vi "CRYSet Limits Run Front Panel.vi"(11 "Vi Ref":refnum<vi>) -> ()   [LabVIEW 2013]
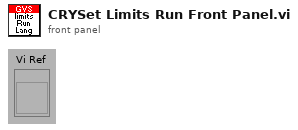
[diagram p1: front panel]
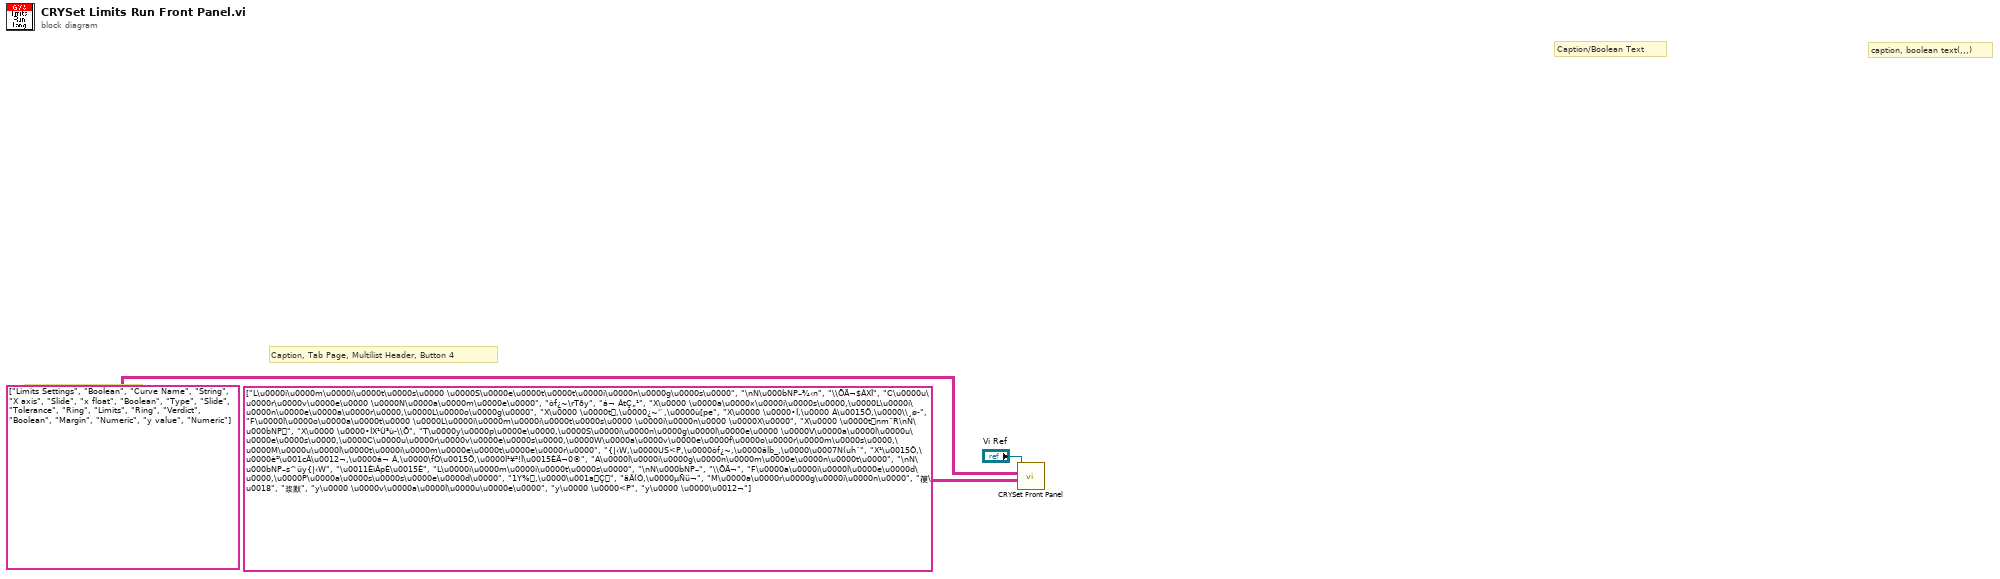
[diagram p0: block diagram]
diagram:
  # "Caption, Tab Page, Multilist Header, Button 4"
  # "Control Type"
  # "Control Name and Tab"
  # "caption, boolean text(,,,)"
  # "Caption/Boolean Text"
  n1 = call "CRYSet Front Panel.vi"("Caption(Boolean Text)"=string[][] [["L\u0000i\u0000m\u0000i\u0000t\u0000s\u0000 \u0000S\u0000e\u0000t\u0000t\u0000i\u0000n\u0000g\u0000s\u0000", "\nN\u000bNP–¾‹n", "\\ÕÄ¬$ÁXÎ"], ["C\u0000u\u0000r\u0000v\u0000e\u0000 \u0000N\u0000a\u0000m\u0000e\u0000", "òf¿~\rTðy", "á¬ ÁtÇ„¹"], ["X\u0000 \u0000a\u0000x\u0000i\u0000s\u0000,\u0000L\u0000i\u0000n\u0000e\u0000a\u0000r\u0000,\u0000L\u0000o\u0000g\u0000", "X\u0000 \u0000t,\u0000¿~'`,\u0000ù[pe", "X\u0000 \u0000•Í,\u0000 Á\u0015Ö,\u0000\\¸ø­"], ["F\u0000l\u0000o\u0000a\u0000t\u0000 \u0000L\u0000i\u0000m\u0000i\u0000t\u0000s\u0000 \u0000i\u0000n\u0000 \u0000X\u0000", "X\u0000 \u0000tnm¨R\nN\u000bNP", "X\u0000 \u0000•ÍX¹Ù³ù­\\Õ"], ["T\u0000y\u0000p\u0000e\u0000,\u0000S\u0000i\u0000n\u0000g\u0000l\u0000e\u0000 \u0000V\u0000a\u0000l\u0000u\u0000e\u0000s\u0000,\u0000C\u0000u\u0000r\u0000v\u0000e\u0000s\u0000,\u0000W\u0000a\u0000v\u0000e\u0000f\u0000o\u0000r\u0000m\u0000s\u0000,\u0000M\u0000u\u0000l\u0000t\u0000i\u0000m\u0000e\u0000t\u0000e\u0000r\u0000", "{|‹W,\u0000US<P,\u0000òf¿~,\u0000âlb_,\u0000\u0007N(uhˆ", "X¹\u0015Ö,\u0000è²\u001cÂ\u0012¬,\u0000á¬ Á,\u0000\fÓ\u0015Ö,\u0000Ì¹¥²!Î\u0015ÈÄ¬0®"], ["A\u0000l\u0000i\u0000g\u0000n\u0000m\u0000e\u0000n\u0000t\u0000", "\nN\u000bNP–s^ûy{|‹W", "\u0011ÉìÂpÈ\u0015È"], ["L\u0000i\u0000m\u0000i\u0000t\u0000s\u0000", "\nN\u000bNP–", "\\ÕÄ¬"], ["F\u0000a\u0000i\u0000l\u0000e\u0000d\u0000,\u0000P\u0000a\u0000s\u0000s\u0000e\u0000d\u0000", "1Y%,\u0000\u001aÇ", "äÂ(Ó,\u0000µÑü¬"], ["M\u0000a\u0000r\u0000g\u0000i\u0000n\u0000", "箯\u0018", "浆默"], ["y\u0000 \u0000v\u0000a\u0000l\u0000u\u0000e\u0000", "y\u0000 \u0000<P", "y\u0000 \u0000\u0012¬"]], "Control ID and Type(Label Name, Type)"=string[][] [["Limits Settings", "Boolean"], ["Curve Name", "String"], ["X axis", "Slide"], ["x float", "Boolean"], ["Type", "Slide"], ["Tolerance", "Ring"], ["Limits", "Ring"], ["Verdict", "Boolean"], ["Margin", "Numeric"], ["y value", "Numeric"]], "Vi Ref"="Vi Ref") -> ()  [unwired: 9 in]
